vi "getRangeInUse_xmlNode.vi"(8 "error in (no error)":errorcluster, 11 "AnalogDevice.lvclass in":refnum<class "AnalogDevice.lvclass">) -> (0 "error out":errorcluster, 2 "rangeInuse_xml":refnum<class "xmlNode.lvclass">, 3 "AnalogDevice.lvclass out":refnum<class "AnalogDevice.lvclass">)   [LabVIEW 2009, in "Tools.lvlib" / "DatabaseHelpers.lvlib" / "AnalogDevice.lvclass"]
uses:
  AnalogDevice.lvclass
  xmlNode/xmlNode.lvclass
  AnalogDevice.lvclass/AnalogDevice.ctl
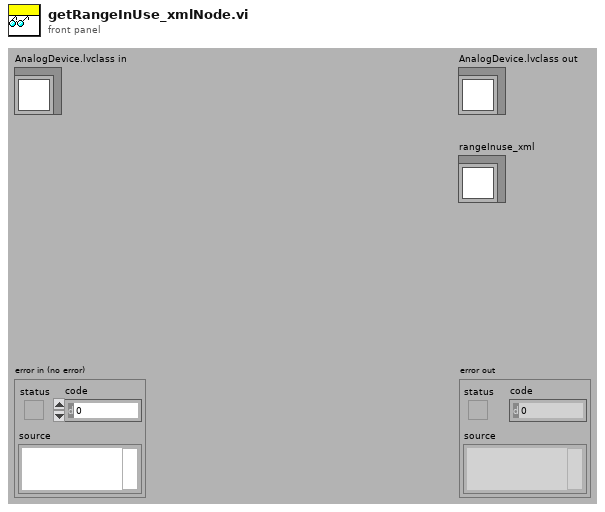
[diagram p1: front panel]
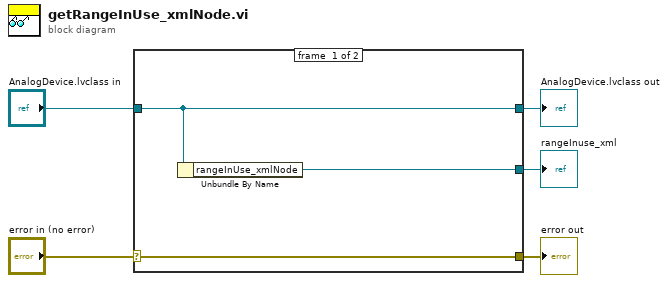
[diagram p0: block diagram]
diagram:
  n1 = case shown="No Error" "error in (no error)" {
    selector: "error in (no error)" -> [w8 w9]
    tunnel: [w8 w9] -> w4
    tunnel: [w7 w10] -> w2
    tunnel: "AnalogDevice.lvclass in" -> [w7 w10]
    tunnel: [w6 _] -> w1
    frame #0 {
      n2 = Unbundle By Name(w7) -> ("rangeInUse_xmlNode"=w6:refnum<class "xmlNode.lvclass">)
    }
    frame #1 {
    }
  }
  "error out" <- w4
  "AnalogDevice.lvclass out" <- w2
  "rangeInuse_xml" <- w1
